vi "Bool to String.vi"(1 "Boolean":bool) -> (0 "String":string)   [LabVIEW 2026, in "TALOS.lvlib"]
doc: "This VI converts \"0\", \"False\", \"FALSE\" and \"false\" to False, and everything else to True."
uses:
  TALOS.lvlib
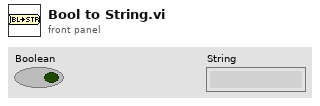
[diagram p1: front panel]
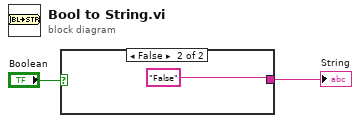
[diagram p0: block diagram]
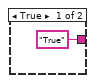
[diagram p2: hidden frame]
diagram:
  n1 = case shown="False" "Boolean" {
    tunnel: ["True" "False"] -> w2
    frame True {
    }
    frame False {
    }
  }
  "String" <- w2
